vi "TBA_NET_Add.vi"(8 "error in (no error)":errorcluster caption="错误输入（无错误）", 9 "Clear First?":bool, 10 "Item[]":T1[](array[typedef]) {"DisplayStyle" items=["None", "Text", "Image", "ImageAndText"]}, 11 "Toolbar Ref":refnum<class "ToolStrip.lvclass">) -> (0 "error out":errorcluster caption="错误输出", 3 "ToolStrip":refnum<class "ToolStrip.lvclass"> caption="Toolbar Ref Out")   [LabVIEW 2016, in "ToolStrip.lvclass"]
uses:
  Pravite/ToolStrip.lvclass
  TBA_NET_Item.ctl
  Pravite/ToolStrip.lvclass/ToolStrip.ctl
  System.Windows.Forms
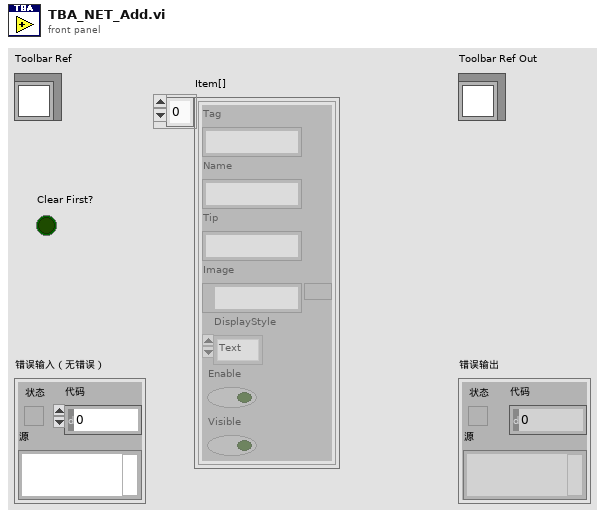
[diagram p1: front panel]
types:
  T1 = typedef "TBA_NET_Item.ctl" = cluster{"Tag":string, "Name":string, "Tip":string, "Image":path, "DisplayStyle":i32, "Enable":bool, "Visible":bool}
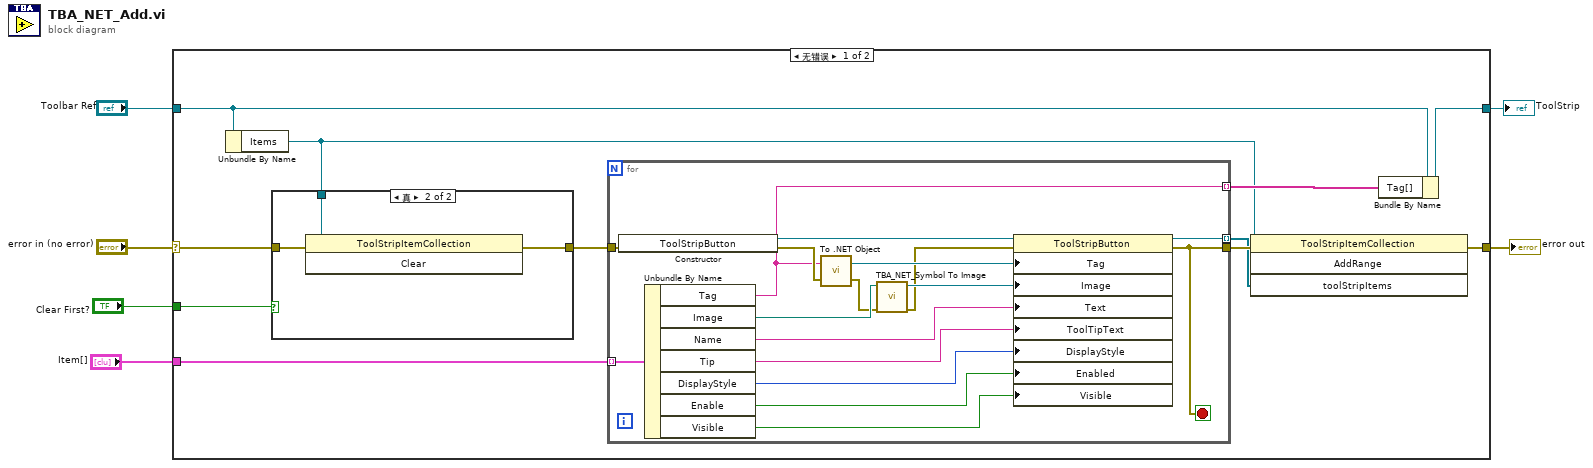
[diagram p0: block diagram]
diagram:
  n1 = case shown="无错误" "error in (no error)" {
    selector: "error in (no error)" -> [w10 w40]
    tunnel: [w14 w40] -> w5
    tunnel: [w12 w39] -> w3
    tunnel: "Toolbar Ref" -> [w13 w39]
    tunnel: "Item[]" -> [w15 _]
    tunnel: "Clear First?" -> [w7 _]
    frame No Error {
      n2 = Unbundle By Name(w13) -> ("Items"=w8:refnum<k24>)
      n3 = case shown="真" w7 {
        tunnel: w10 -> [w18 w21]
        tunnel: [w18 w20] -> w9
        tunnel: w8 -> [_ w19]
        frame False {
        }
        frame True {
          n4 = invoke class="ToolStripItemCollection" method="Clear"(reference=w19, error in=w21) -> (error out=w20:errorcluster)  [unwired: 1 in, 2 out]
        }
      }
      n5 = for {
        tunnel: w15 -> [w34] mode=indexing
        tunnel: [w36] -> w16 mode=indexing
        tunnel: w9 -> [w35]
        tunnel: [w22] -> w17
        tunnel: [w23] -> w11 mode=indexing
        stop <- w22 stop-if-true
        n6 = constructor class="ToolStripButton"(error in=w35) -> (reference out=w37:refnum<k24>, error out=w33:errorcluster)  [unwired: 2 in, 1 out]
        n7 = Unbundle By Name(w34) -> ("Tag"=w23:string, "Image"=w30:path, "Name"=w31:string, "Tip"=w32:string, "DisplayStyle"=w26:i32, "Enable"=w25:bool, "Visible"=w24:bool)
        n8 = call <vilib>:"To .NET Object.vi"("error in (no error)"=w33, "anything"=w23) -> ("error out"=w29:errorcluster, ".NET object"=w38:refnum<k24>)
        n9 = call "TBA_NET_Symbol To Image.vi"("Error In"=w29, "IconPath"=w30) -> ("Error Out"=w27:errorcluster, "Image"=w28:refnum<k24>)  [unwired: 8 in]
        n10 = property class="ToolStripButton"(reference=w37, error in=w27, "Tag"=w38, "Image"=w28, "Text"=w31, "ToolTipText"=w32, "DisplayStyle"=w26, "Enabled"=w25, "Visible"=w24) -> (reference out=w36:refnum<k24>, error out=w22:errorcluster)
      }
      n11 = invoke class="ToolStripItemCollection" method="AddRange"(reference=w8, error in=w17, "toolStripItems"=w16) -> (error out=w14:errorcluster)  [unwired: 1 in, 3 out]
      n12 = Bundle By Name(cluster=w13, "Tag[]"=w11) -> (w12:refnum<class "ToolStrip.lvclass">)
    }
    frame Error {
    }
  }
  "error out" <- w5
  "ToolStrip" <- w3
